vi "SIM Calculate Machine Epsilon.vi"() -> (0 "min float":dbl, 1 "machine eps":dbl)   [LabVIEW 2017]
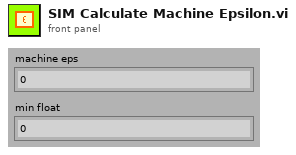
[diagram p1: front panel]
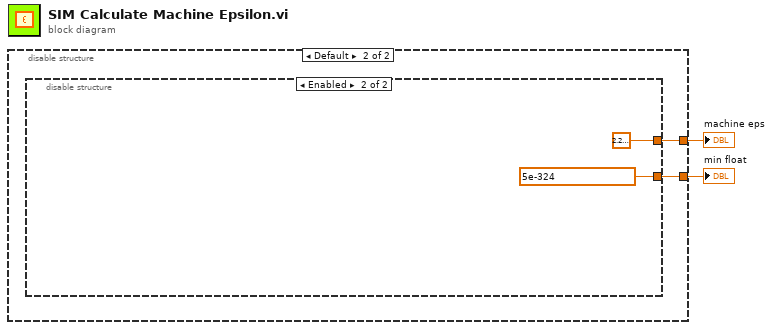
[diagram p0: block diagram]
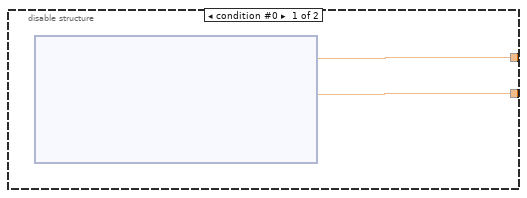
[diagram p2: hidden frame]
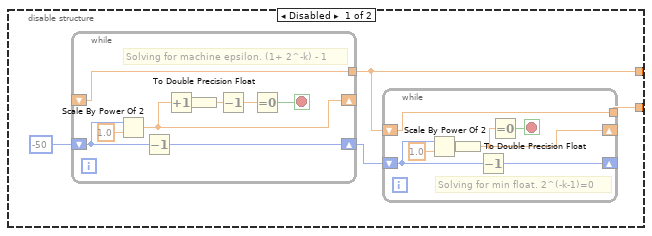
[diagram p3: hidden frame]
diagram:
  n1 = disable-structure shown="Default" {
    disable-tunnel: [w4 w6] -> w2
    disable-tunnel: [w3 w5] -> w1
    frame condition #0 {
      n2 = node() -> (w4:dbl, w3:dbl)
    }
    frame condition #1 (active) {
      n3 = disable-structure shown="Enabled" {
        disable-tunnel: [w8 2.220446049250313e-16] -> w6
        disable-tunnel: [w7 5e-324 ("min float")] -> w5
        frame Disabled {
          n4 = while {
            shift-right: [w23] -> w10
            shift-left: -50 -> [w20]
            shift-right: [w19] -> _
            shift-left: _ -> [w22]
            tunnel: [w22] -> w8
            stop <- w26 stop-if-true
            # "Solving for machine epsilon. (1+ 2^-k) - 1"
            n5 = Scale By Power Of 2(n=w20, x=1.0) -> (x*2^n=w19:dbl)
            n6 = Decrement(x=w20) -> (x-1=w23:i32)
            n7 = Increment(x=w19) -> (x+1=w25:dbl)
            n8 = To Double Precision Float(number=w25) -> (double precision float=w18:dbl)
            n9 = Decrement(x=w18) -> (x-1=w24:dbl)
            n10 = Equal To 0?(x=w24) -> (x = 0?=w26:bool)
          }
          n11 = while {
            shift-right: [w14] -> _
            shift-left: w10 -> [w15]
            shift-right: [w11] -> _
            shift-left: w8 -> [w17]
            tunnel: [w17] -> w7
            stop <- w13 stop-if-true
            # "Solving for min float. 2^(-k-1)=0"
            n12 = Scale By Power Of 2(n=w15, x=1.0) -> (x*2^n=w12:dbl)
            n13 = To Double Precision Float(number=w12) -> (double precision float=w11:dbl)
            n14 = Decrement(x=w15) -> (x-1=w14:i32)
            n15 = Equal To 0?(x=w11) -> (x = 0?=w13:bool)
          }
        }
        frame Enabled {
        }
      }
    }
  }
  "machine eps" <- w2
  "min float" <- w1
